vi "Get Units.vi"(3 "WavBuf":refnum<class "WavBuf.lvclass">) -> (1 "Units Out":string)   [LabVIEW 2024, in "WavBuf.lvclass"]
uses:
  WavBuf.lvclass
  WavBuf.lvclass/WavBuf.ctl
  Universal Controls/Read Write Button.ctl
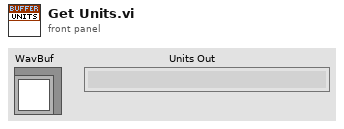
[diagram p1: front panel]
types:
  T1 = typedef "Ref_DVR_Buffer.ctl" = refnum<data-value>
  T2 = typedef "Read Write Button.ctl" = bool
  T3 = typedef "Waveform_Data.ctl" = waveform(dbl)
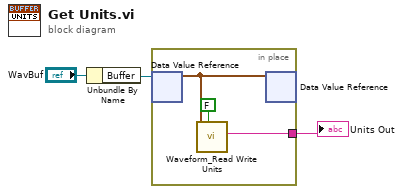
[diagram p0: block diagram]
diagram:
  n1 = Unbundle By Name("WavBuf") -> ("Buffer"=w2:T1)
  n2 = in-place {
    in-place-border: [w5] -> w1
    n3 = in-place-dvr #1(w2) -> (w6:T3)  [unwired: 1 out]
    n4 = call "Waveform_Read Write Units.vi"("Read(f)\nWrite(t)"=T2 FALSE ("Read(f)\nWrite(t)"), "Raw Data Waveform"=w6) -> ("Name Out"=w5:string)  [unwired: 8 in, 1 out]
    n5 = in-place-dvr #1(w6) -> ()  [unwired: 2 out]
  }
  "Units Out" <- w1
